vi "Untitled 14.vi"() -> ()   [LabVIEW 2009]
uses:
  Dryer.ctl
  Dryer Details.ctl
panel:
  out "Numeric":i32
  out "Boolean 2":bool
  in  "Boolean":bool
  in  "Color Box 2":u32(colorbox)
  in  "output array":T1[](array[typedef]) {"Station Number" format="%02.0f"; "Cycle Count" format="%0#4_4g"}
  in  "Dryer":T1 {"Station Number" format="%02.0f"; "Cycle Count" format="%0#4_4g"}
  in  "GUI Aisle 1":T1[](array[typedef]) {"Station Number" format="%02.0f"; "Cycle Count" format="%0#4_4g"}
  in  "Color Box":u32(colorbox)
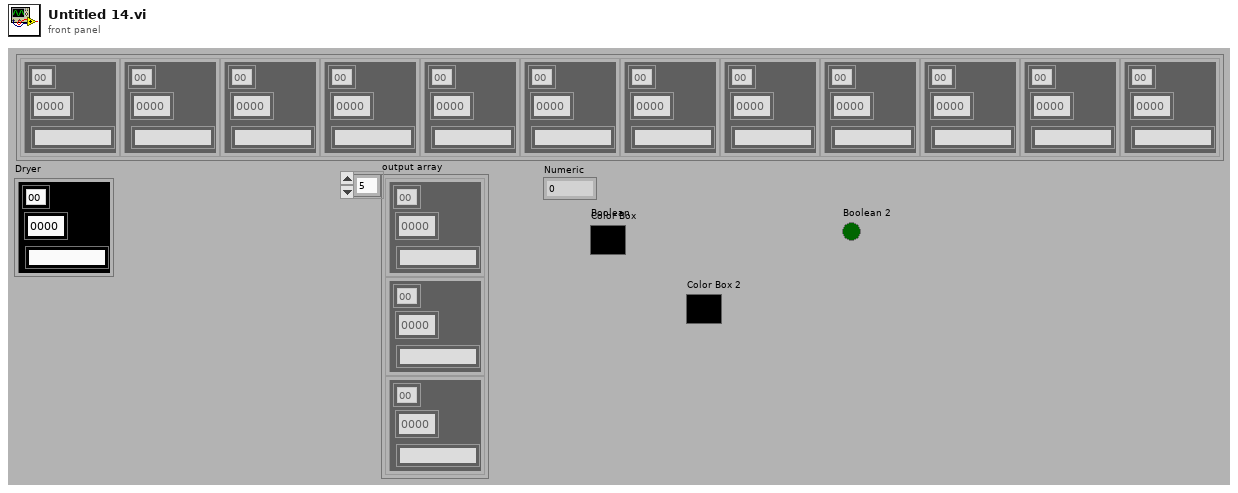
[diagram p1: front panel]
types:
  T1 = typedef "Dryer.ctl" = cluster{"Serial Number":string, "Cycle Count":dbl, "Station Number":u8, "Dryer Details":T2, "Sample Record(t, Cycle Count, t-cum,L1, L2, V, Trmb, ASCII, Status) ":string[][], "Hist Record(Cycle Count, t-comp,L1max, L2max, Tmax) ":string[][], "Status Color":u32, "Boolean":bool}
  T2 = typedef "Dryer Details.ctl" = cluster{"Station":string, "Cycle Count":string, "Status":string, "Debug ASCII":string, "Note":string, "FILEMNAME":string, "Serial Number":string, "Total Time Drying":string}
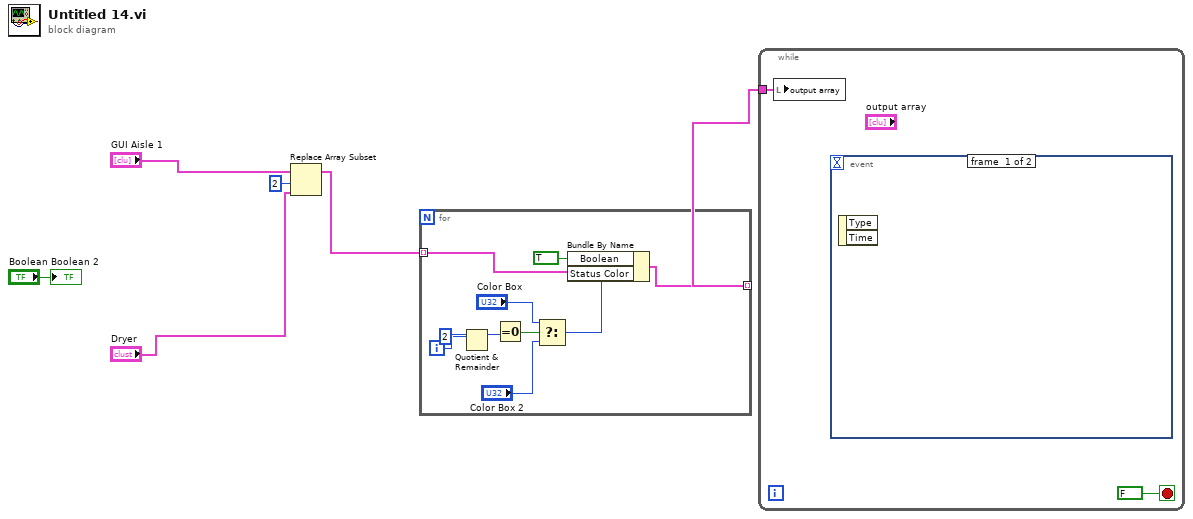
[diagram p0: block diagram]
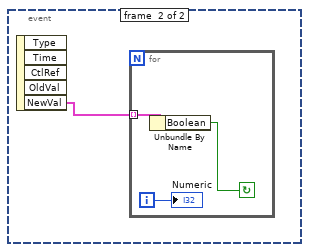
[diagram p2: hidden frame]
diagram:
  n1 = Replace Array Subset(array="GUI Aisle 1", new element="Dryer", index=2) -> (w3:T1[])
  n2 = for {
    tunnel: w3 -> [w10] mode=indexing
    tunnel: [w8] -> w1 mode=indexing
    i -> [w16]
    n3 = Quotient & Remainder(x=w16, y=2) -> (x-y*floor(x/y)=w14:i32)  [unwired: 1 out]
    n4 = Equal To 0?(x=w14) -> (x = 0?=w13:bool)
    n5 = Select(t="Color Box", s=w13, f="Color Box 2") -> (s? t:f=w9:u32)
    n6 = Bundle By Name(cluster=w10, "Boolean"=TRUE, "Status Color"=w9) -> (w8:T1)
  }
  n7 = while {
    tunnel: w1 -> [w18]
    stop <- FALSE stop-if-true
    n8 = local write "output array"(w18) -> ()
    n9 = event shown="[1] \"output array\": Value Change" {
      selector: _ -> [_ _]
      dyn-events: _ -> [_ _]
      timeout: _ -> [_ _]
      event #0 {
        n10 = event-data() -> ()  [unwired: 1 in, 2 out]
      }
      event #1 {
        n11 = event-data() -> ("NewVal"=w19:T1[])  [unwired: 1 in, 4 out]
        n12 = for {
          tunnel: w19 -> [w20] mode=indexing
          i -> [w21]
          stop <- w22 continue-if-true
          n13 = Unbundle By Name(w20) -> ("Boolean"=w22:bool)
          "Numeric" <- w21
        }
      }
    }
  }
  "Boolean 2" <- "Boolean"
